vi "FG Motor Instruction.vi"(1 "FG Action (Read)":T4, 2 "Motor Instruction in":T1={"Motor State"=enum."Stop", "Motor Command"={"Speed"=0, "Turn"=0}}) -> (0 "Motor Instruction out":T1={"Motor State"=enum."Stop", "Motor Command"={"Speed"=0, "Turn"=0}})   [LabVIEW 2009]
uses:
  Actions for FG's.ctl
  Remote Control/Motor Command.ctl
  Queue Type Def's/Motor State.ctl
  Queue Type Def's/Motor Instruction.ctl
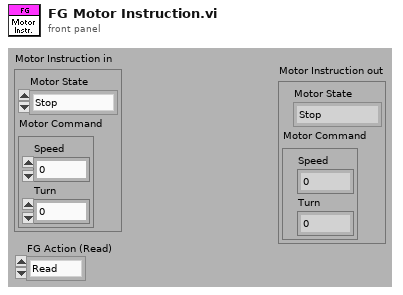
[diagram p1: front panel]
types:
  T1 = typedef "Motor Instruction.ctl" = cluster{"Motor State":T2, "Motor Command":T3}
  T2 = typedef "Motor State.ctl" = enum16{"Wait", "Initialize", "Check FET", "Run", "Stop"}
  T3 = typedef "Motor Command.ctl" = cluster{"Speed":i16, "Turn":i16}
  T4 = typedef "Actions for FG's.ctl" = enum16{"Read", "Write"}
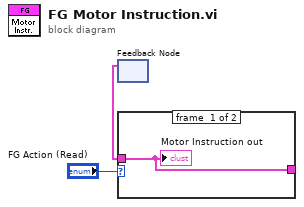
[diagram p0: block diagram]
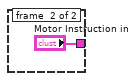
[diagram p2: hidden frame]
diagram:
  n1 = feedback #1() -> (w3:T1)  [unwired: 1 in]
  n2 = case shown="\"Read\", Default" "FG Action (Read)" {
    tunnel: [w4 "Motor Instruction in"] -> w2
    tunnel: w3 -> [w4 _]
    frame #0 {
      "Motor Instruction out" <- w4
    }
    frame #1 {
    }
  }
